vi "Main.vi"(8 "error in":errorcluster caption="entrée d'erreur") -> (0 "error out":errorcluster caption="sortie d'erreur")   [LabVIEW 2026]
uses:
  <vilib>/DAQmx/read.llb/DAQmx Read (Analog 1D DBL 1Chan NSamp).vi
  <vilib>/DAQmx/read.llb/DAQmx Read (Counter 1D DBL 1Chan NSamp).vi
  <vilib>/DAQmx/miscellaneous.llb/DAQmx Fill In Error Info.vi
panel:
  in  "MAIN stop":bool
  in  "Start":bool
  in  "Dwell time (µs)":dbl=2.0 format="%#_13g"
  out "PMT_Scan":dbl[][](graph)
  out "PMT_i(t)":waveform(dbl)(graph)
  out "APD_i(t)":waveform(dbl)(graph)
  out "APD_Scan":dbl[][](graph)
  in  "Stop":bool
  in  "Continuous?":bool
  in  "Scan XY (T) / i(t) (F)":bool
  in  "Position XY (for i(t))":dbl[](array[numeric])=[5.0, 5.0]
  in  "Scanning cluster":T1={"Nx"=4, "Ny"=4, "# Repetition"=1, "FOV_X (µm)"=100.0, "FOV_Y (µm)"=100.0, "Calib_X"=0.1, "Calib_Y"=0.1, "Center X (µm)"=50.0, "Center_Y (µm)"=50.0, "Bi-directionnal?"=FALSE} {"# Repetition" min=1 step=1; "Ny" min=1 step=1; "Nx" min=1 step=1}
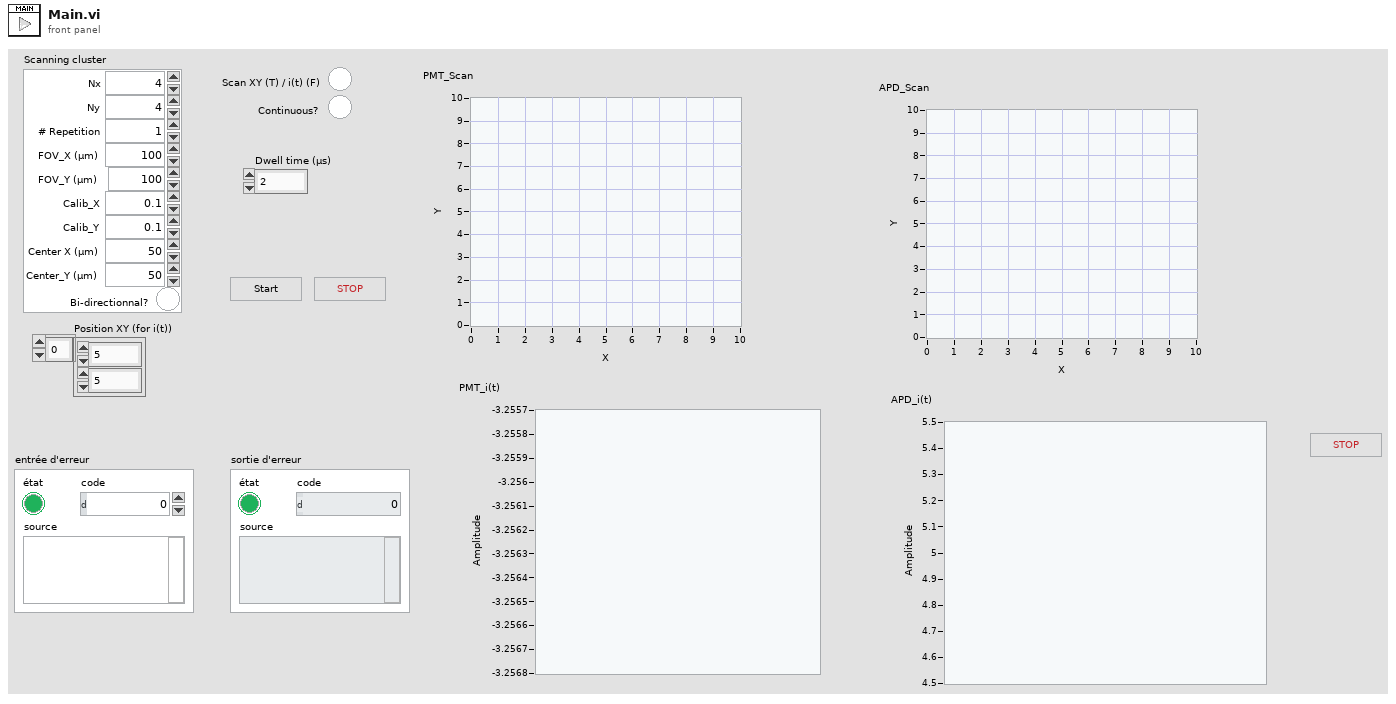
[diagram p1: front panel]
types:
  T1 = cluster{"Nx":u16, "Ny":u16, "# Repetition":u16, "FOV_X (µm)":dbl, "FOV_Y (µm)":dbl, "Calib_X":dbl, "Calib_Y":dbl, "Center X (µm)":dbl, "Center_Y (µm)":dbl, "Bi-directionnal?":bool}
  T2 = cluster{"CO task":refnum<k21>, "AO task":refnum<k21>, "AI task":refnum<k21>, "CI task":refnum<k21>}
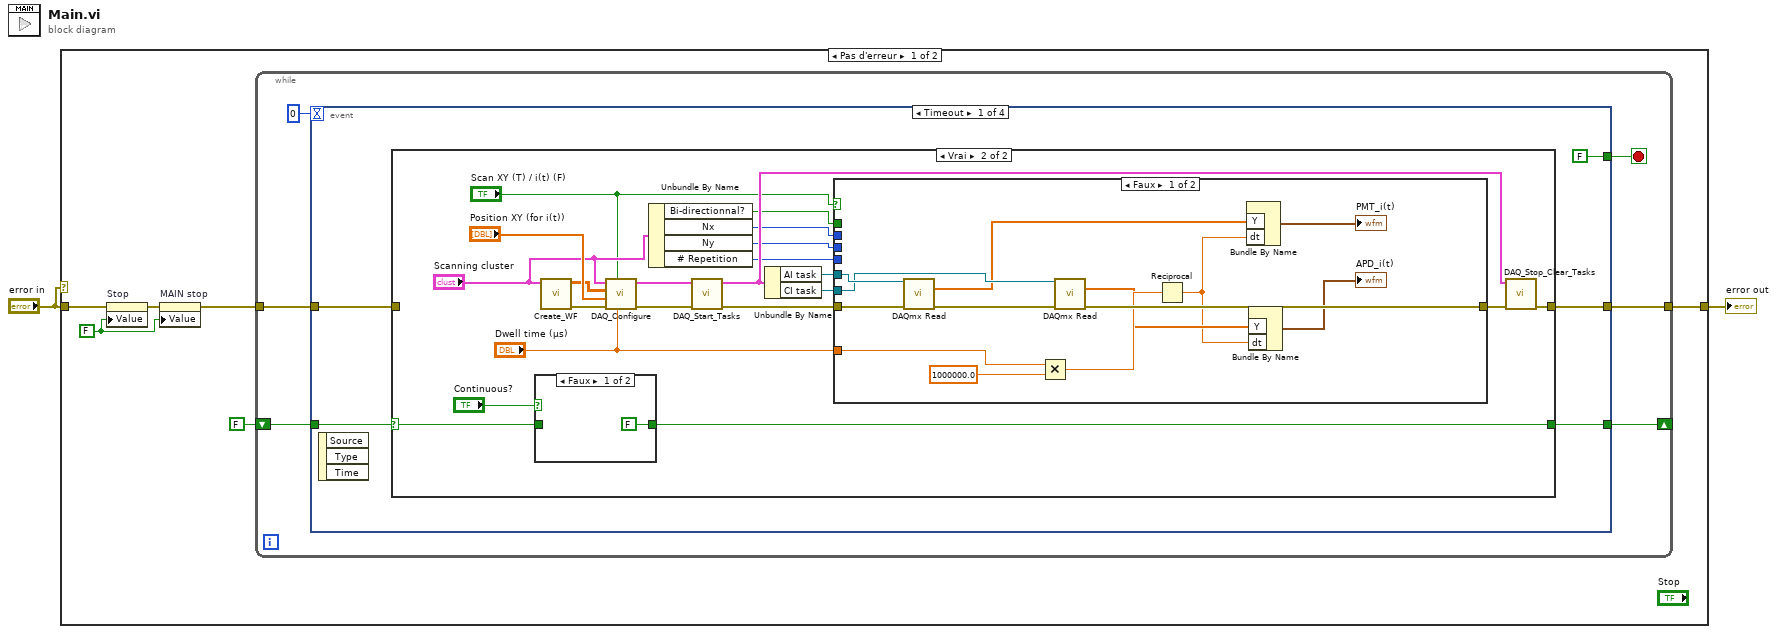
[diagram p0: block diagram]
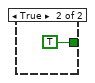
[diagram p3: hidden frame]
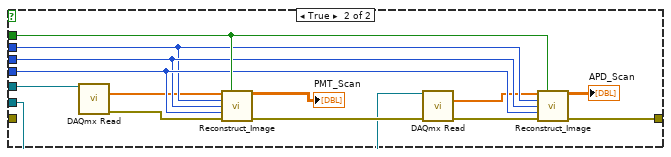
[diagram p4: hidden frame]
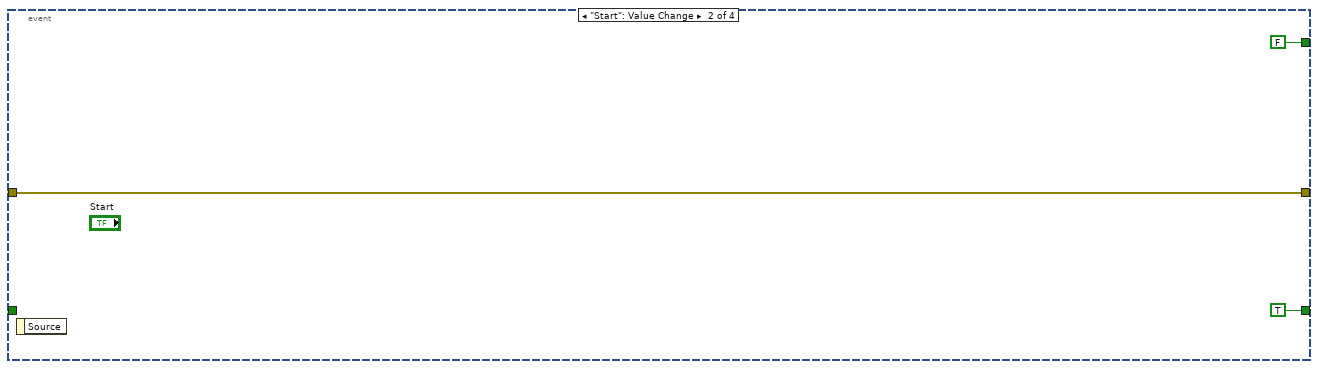
[diagram p5: hidden frame]
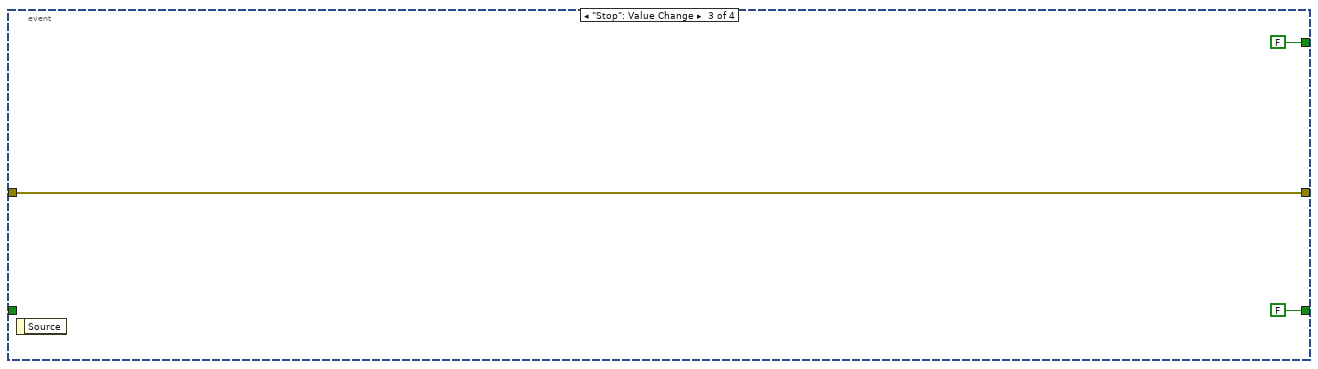
[diagram p6: hidden frame]
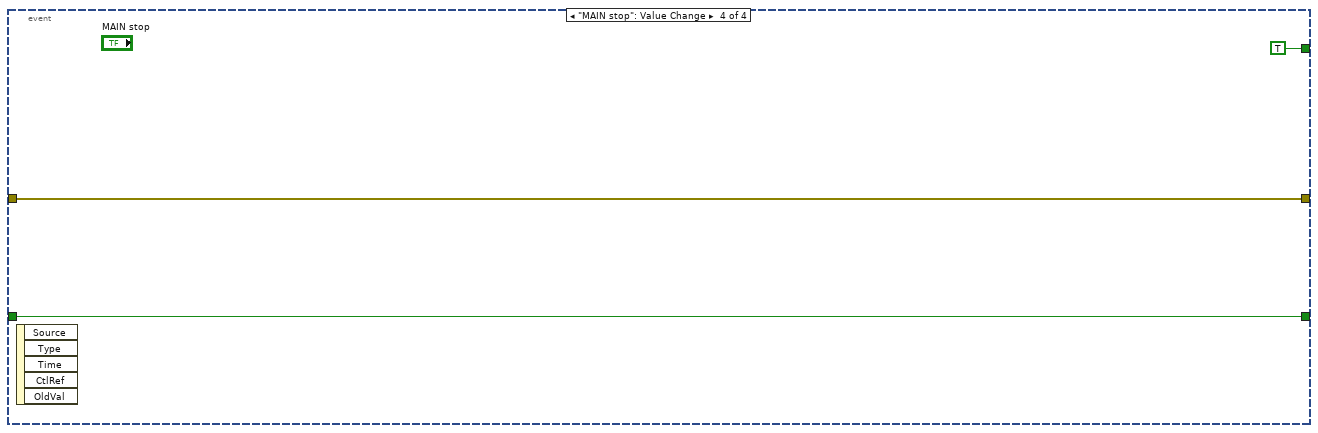
[diagram p7: hidden frame]
diagram:
  n1 = case shown="Pas d'erreur" "error in" {
    selector: "error in" -> [_ w81]
    tunnel: [w7 w81] -> w2
    tunnel: "error in" -> [w6 _]
    frame No Error {
      w5 = FALSE ("Stop")
      n2 = property on="Stop" class="Bool"(error in=w6, "Value"=w5) -> (error out=w4:errorcluster)  [unwired: 1 in, 1 out]
      n3 = property on="MAIN stop" class="Bool (strict)"(error in=w4, "Value"=w5) -> (error out=w3:errorcluster)  [unwired: 1 in, 1 out]
      n4 = while {
        shift-right: [w13] -> _
        shift-left: FALSE -> [w12]
        tunnel: w3 -> [w10]
        tunnel: [w9] -> w7
        stop <- w11 stop-if-true
        n5 = event shown="[0] Timeout" {
          selector: _ -> [_ _ _ _]
          dyn-events: _ -> [_ _ _ _]
          timeout: 0 -> [_ _ _ _]
          tunnel: [w15 TRUE FALSE w78] -> w13
          tunnel: w12 -> [w16 _ _ w78]
          tunnel: [FALSE ("NewVal") FALSE ("NewVal") FALSE ("NewVal") TRUE ("NewVal")] -> w11
          tunnel: w10 -> [w17 w73 w76 w80]
          tunnel: [w18 w73 w76 w80] -> w9
          event Timeout {
            n6 = event-data() -> ()  [unwired: 1 in, 3 out]
            n7 = case shown="Vrai" w16 {
              selector: w16 -> [w20 w25]
              tunnel: [w21 w26] -> w18
              tunnel: w17 -> [w21 _]
              tunnel: [w20 w23] -> w15
              frame False {
              }
              frame True {
                n8 = case shown="Faux" "Continuous?" {
                  tunnel: w25 -> [_ _]
                  tunnel: [FALSE TRUE] -> w23
                  frame False {
                  }
                  frame True {
                  }
                }
                n9 = call "Create_WF.vi"("Scanning cluster"="Scanning cluster") -> ("error out"=w31:errorcluster, "Scanning positions"=w32:dbl[][])  [unwired: 8 in, 1 out]
                n10 = call "DAQ_Configure.vi"("Dwell time (µs)"="Dwell time (µs)", "Scan XY (T) / i(t) (F)"="Scan XY (T) / i(t) (F)", "error in"=w31, "Position XY (for i(t))"="Position XY (for i(t))", "Scanning positions"=w32, "Scanning cluster"="Scanning cluster") -> ("error out"=w27:errorcluster, "Task cluster"=w29:T2)  [unwired: 4 in]
                n11 = Unbundle By Name("Scanning cluster") -> ("Bi-directionnal?"=w34:bool, "Nx"=w35:u16, "Ny"=w36:u16, "# Repetition"=w37:u16)
                n12 = call "DAQ_Start_Tasks.vi"("entrée d'erreur (pas d'erreur)"=w27, "Task cluster"=w29) -> ("sortie d'erreur"=w38:errorcluster, "Task cluster OUT"=w42:T2)  [unwired: 8 in]
                n13 = Unbundle By Name(w42) -> ("AI task"=w39:refnum<k21>, "CI task"=w40:refnum<k21>)
                n14 = case shown="Faux" "Scan XY (T) / i(t) (F)" {
                  tunnel: w34 -> [_ w70]
                  tunnel: w35 -> [_ w67]
                  tunnel: w36 -> [_ w68]
                  tunnel: w37 -> [_ w69]
                  tunnel: [w56 w62] -> w41
                  tunnel: w38 -> [w55 _]
                  tunnel: w39 -> [w54 w59]
                  tunnel: w40 -> [w53 w58]
                  tunnel: "Dwell time (µs)" -> [w49 _]
                  frame False {
                    n15 = call-poly <vilib>:"DAQmx Read.vi"("task/channels in"=w54, "error in"=w55) -> ("data"=w52:dbl[], "error out"=w57:errorcluster)  [unwired: 11 in, 1 out]
                    n16 = Multiply(x=w49, y=1000000.0) -> (x*y=w48:dbl)
                    n17 = call-poly <vilib>:"DAQmx Read.vi"("task/channels in"=w53, "error in"=w57) -> ("data"=w47:dbl[], "error out"=w56:errorcluster)  [unwired: 11 in, 1 out]
                    n18 = Reciprocal(x=w48) -> (1/x=w45:dbl)
                    n19 = Bundle By Name("Y"=w52, "dt"=w45) -> (→"PMT_i(t)":waveform(dbl))  [unwired: 1 in]
                    n20 = Bundle By Name("Y"=w47, "dt"=w45) -> (→"APD_i(t)":waveform(dbl))  [unwired: 1 in]
                  }
                  frame True {
                    n21 = call-poly <vilib>:"DAQmx Read.vi"("task/channels in"=w59) -> ("data"=w65:dbl[], "error out"=w66:errorcluster)  [unwired: 12 in, 1 out]
                    n22 = call "Reconstruct_Image.vi"("Data_AI"=w65, "Bidirectionnel?"=w70, "Nx"=w67, "Ny"=w68, "# Repetition"=w69, "error in"=w66) -> ("Channel 1"=→"PMT_Scan":dbl[][], "error out"=w71:errorcluster)  [unwired: 7 in, 1 out]
                    n23 = call-poly <vilib>:"DAQmx Read.vi"("task/channels in"=w58, "error in"=w71) -> ("data"=w64:dbl[], "error out"=w63:errorcluster)  [unwired: 11 in, 1 out]
                    n24 = call "Reconstruct_Image.vi"("Data_AI"=w64, "Bidirectionnel?"=w70, "Nx"=w67, "Ny"=w68, "# Repetition"=w69, "error in"=w63) -> ("Channel 1"=→"APD_Scan":dbl[][], "error out"=w62:errorcluster)  [unwired: 7 in, 1 out]
                  }
                }
                n25 = call "DAQ_Stop_Clear_Tasks.vi"("error in"=w41, "Cluster tasks"=w42) -> ("sortie d'erreur"=w26:errorcluster)  [unwired: 9 in]
              }
            }
          }
          event "Start": Value Change {
            n26 = event-data() -> ()  [unwired: 1 in, 1 out]
          }
          event "Stop": Value Change {
            n27 = event-data() -> ()  [unwired: 1 in, 1 out]
          }
          event "MAIN stop": Value Change {
            n28 = event-data() -> ()  [unwired: 1 in, 5 out]
          }
        }
      }
    }
    frame Error {
    }
  }
  "error out" <- w2
